vi "Test App Get All Processes.vi"(8 "error in (no error)":errorcluster, 11 "Rig Test in":refnum<class "Application Test.lvclass">) -> (0 "error out":errorcluster, 3 "Rig Test out":refnum<class "Application Test.lvclass">)   [LabVIEW 2020, in "Application Test.lvclass"]
uses:
  Application Test.lvclass
  C:/Program Files (x86)/National Instruments/LabVIEW 2020/vi.lib/Astemes/LUnit/Test Case.lvclass
  Framework/Process/Process.lvclass
  Framework/Process/Process.lvclass/Process.ctl
  Framework/Application/Application.lvclass/Application.ctl
  <vilib>/Astemes/LUnit/Test Case.lvclass/Test Case.ctl
  <vilib>/Astemes/LUnit/LUnit Assertion Result.lvclass/LUnit Assertion Result.ctl
  <vilib>/Astemes/LUnit/LUnit Test Case Result.lvclass/LUnit Test Case Result.ctl
  <vilib>/Astemes/LUnit/LUnit Method Result.lvclass/LUnit Method Result.ctl
  6f2e4378-1cf5-42ff-8d03-6273ee4332bb.vi
  Framework/Process/Public/Lifecycle/Get Lifecycle State.vi
  Framework/Process/Protected/Messaging/Request Message.vi
  Framework/Application/Private/Add Process to Map.vi
  Framework/Application/Private/Start Idle Processes if Running.vi
  Framework/Application/Private/Throw Error If Process Already in App.vi
  Framework/Process/Protected/Messaging/Enqueue Message.vi
  Framework/Process/Protected/SubVIs/Set Context.vi
  <vilib>/Astemes/LUnit/Palette/Pass.vi
  <vilib>/Astemes/LUnit/Palette/Fail.vi
  <vilib>/Astemes/LUnit/Compare Variants.vi
  <vilib>/Astemes/LUnit/Describe Comparison.vi
  <vilib>/Astemes/LUnit/Set Assertion Type.vi
  Framework/Process/Private/SubVIs/Wait for finish.vi
  Framework/Process/Private/SubVIs/Set Lifecycle State.vi
  <vilib>/Utility/error.llb/Clear Errors.vi
  Framework/Process/Private/SubVIs/Handle Debug Data.vi
  Framework/Process/Private/SubVIs/Enqueue Request Message.vi
  Framework/Application/Public/Get Process.vi
  Framework/Process/Public/Lifecycle/Leave Process Loop.vi
  <vilib>/Astemes/LUnit/Add test result.vi
  <vilib>/Astemes/LUnit/LUnit Write Passed.vi
  <vilib>/Astemes/LUnit/LUnit Write Message.vi
  <vilib>/Astemes/LUnit/LUnit Write Description.vi
  <vilib>/Astemes/LUnit/Variant to string.vi
  <vilib>/Astemes/LUnit/LUnit Write Assertion Type.vi
  Framework/Logging/Log Debug.vi
  <vilib>/AdvancedString/1D String Array to Delimited String.vi
  <vilib>/Utility/High Resolution Relative Seconds.vi
  Framework/Application/Private/Retrieve Process from App.vi
  Framework/Application/Private/Parse Process Name.vi
  Framework/Application/Private/Get Process from Map.vi
  <vilib>/Astemes/LUnit/LUnit Record Assertion Result.vi
  <vilib>/AdvancedString/Delimited String to 1D String Array.vi
  <vilib>/Astemes/LUnit/LUnit Aggregate Assertion Results.vi
  <vilib>/Astemes/LUnit/Assertion Result/LUnit Read Status.vi
  <vilib>/Astemes/LUnit/LUnit Read Message.vi
  <vilib>/Astemes/LUnit/LUnit Read Description.vi
  <vilib>/Astemes/LUnit/Method Result/LUnit Merge Status.vi
  <vilib>/Astemes/LUnit/LUnit Concatenate result strings.vi
  Framework/Application/Application.lvclass
  C:/Git/astemes-triarc-framework/source/Framework/Process/Process.lvclass
  <vilib>/Utility/error.llb/Error Cluster From Error Code.vi
  Framework/Process/Public/Read Name.vi
  Framework/Process/Private/SubVIs/Wait for Response Message.vi
  <vilib>/Utility/Data Type/Get Type Information.vi
  <vilib>/Utility/LVClass/Get LV Class Name.vi
  <vilib>/Astemes/LUnit/LUnit Assertion Result.lvclass
  Application Test.lvclass/Application Test.ctl
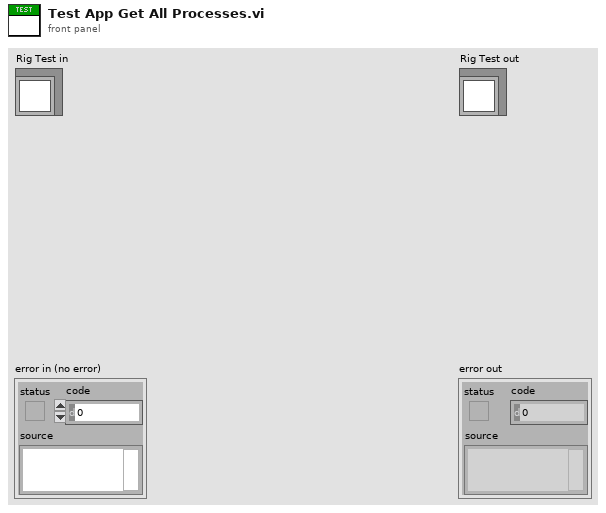
[diagram p1: front panel]
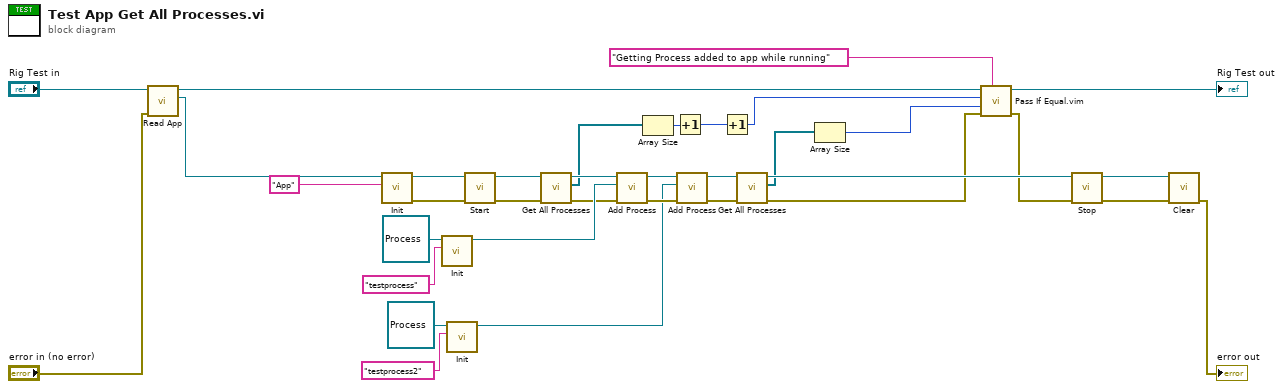
[diagram p0: block diagram]
diagram:
  n1 = call "Read App.vi"("error in (no error)"="error in (no error)", "Application Test In"="Rig Test in") -> ("App out"=w34:refnum<class "Application.lvclass">, "Application Test Out"=w22:refnum<class "Application Test.lvclass">)  [unwired: 7 in, 1 out]
  n2 = call-dynamic "Init.vi"("Name"="App", "Process In"=w34) -> ("error out"=w23:errorcluster, "Process Out"=w24:refnum<class "Application.lvclass">)  [unwired: 8 in]
  n3 = call-dynamic "Init.vi"("Name"="testprocess", "Process In"=refnum<class "Process.lvclass"> refnum ("Process.lvclass")) -> ("Process Out"=w21:refnum<class "Process.lvclass">)  [unwired: 8 in, 1 out]
  n4 = call-dynamic "Init.vi"("Name"="testprocess2", "Process In"=refnum<class "Process.lvclass"> refnum ("Process.lvclass")) -> ("Process Out"=w8:refnum<class "Process.lvclass">)  [unwired: 8 in, 1 out]
  n5 = call "Start.vi"("error in (no error)"=w23, "Process In"=w24) -> ("error out"=w25:errorcluster, "Process Out"=w6:refnum<class "Application.lvclass">)  [unwired: 7 in, 1 out]
  n6 = call "Get All Processes.vi"("error in (no error)"=w25, "Application In"=w6) -> ("error out"=w7:errorcluster, "App Processes"=w1:refnum<class "Process.lvclass">[], "Application Out"=w5:refnum<class "Application.lvclass">)  [unwired: 7 in]
  n7 = call "Add Process.vi"("error in (no error)"=w7, "Process"=w21, "Application In"=w5) -> ("error out"=w29:errorcluster, "Application Out"=w15:refnum<class "Application.lvclass">)  [unwired: 7 in]
  n8 = Array Size(array=w1) -> (size(s)=w2:i32)
  n9 = Increment(x=w2) -> (x+1=w4:i32)
  n10 = call "Add Process.vi"("error in (no error)"=w29, "Process"=w8, "Application In"=w15) -> ("error out"=w16:errorcluster, "Application Out"=w14:refnum<class "Application.lvclass">)  [unwired: 7 in]
  n11 = Increment(x=w4) -> (x+1=w3:i32)
  n12 = call "Get All Processes.vi"("error in (no error)"=w16, "Application In"=w14) -> ("error out"=w12:errorcluster, "App Processes"=w11:refnum<class "Process.lvclass">[], "Application Out"=w32:refnum<class "Application.lvclass">)  [unwired: 7 in]
  n13 = Array Size(array=w11) -> (size(s)=w10:i32)
  n14 = call "Pass If Equal.vim"("Description"="Getting Process added to app while running", "error in (no error)"=w12, "Actual"=w10, "Expected"=w3, "LUnit Test Case In"=w22) -> ("error out"=w27:errorcluster, "LUnit Test Case Out"=→"Rig Test out":refnum<class "Application Test.lvclass">)  [unwired: 5 in]
  n15 = call "Stop.vi"("error in (no error)"=w27, "Process In"=w32) -> ("error out"=w19:errorcluster, "Process Out"=w18:refnum<class "Application.lvclass">)  [unwired: 7 in, 1 out]
  n16 = call-dynamic "Clear.vi"("error in (no error)"=w19, "Application In"=w18) -> ("error out"=→"error out":errorcluster)  [unwired: 9 in]
